vi "OPEN NEW WORKBOOK.vi"(2 "错误输入（无错误）":errorcluster, 3 "Filename":string, 4 "Excel._Application":refnum<k7>) -> (0 "错误输出":errorcluster, 1 "Excel._Application 2":refnum<k7>)   [LabVIEW 2018]
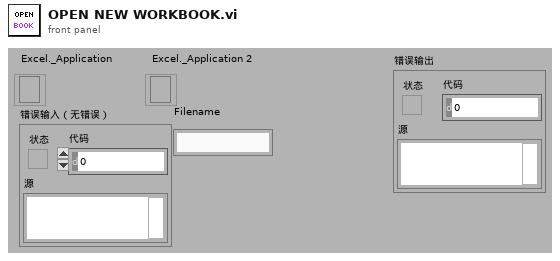
[diagram p1: front panel]
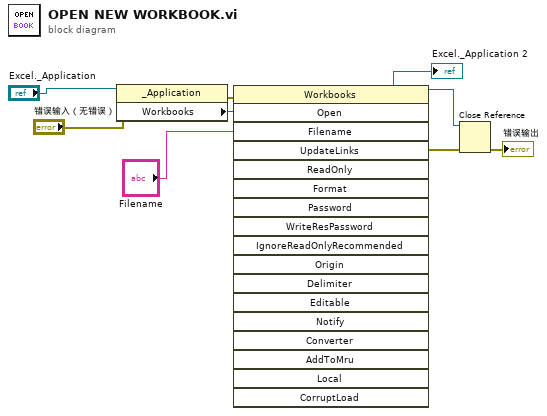
[diagram p0: block diagram]
diagram:
  n1 = property class="_Application"(reference="Excel._Application", error in="错误输入（无错误）") -> (error out=w7:errorcluster, "Workbooks"=w6:refnum<k7>)  [unwired: 1 out]
  n2 = invoke class="Workbooks" method="Open"(reference=w6, error in=w7, "Filename"="Filename") -> (reference out=w4:refnum<k7>, error out=w3:errorcluster, "Open"=→"Excel._Application 2":refnum<k7>)  [unwired: 15 in, 15 out]
  n3 = Close Reference(reference=w4, error in (no error)=w3) -> (error out=→"错误输出":errorcluster)
